vi "Symphony Init.vi"(7 "error In":errorcluster, 9 "Unique id:":string="CCD100", 10 "JYCCDLib.IJYCCDReqd":refnum<k7>) -> (0 "error out":errorcluster, 1 "activeYPixels":i32=256, 2 "activeXPixels":i32=1024, 3 "JYCCDLib.IJYCCDReqd":refnum<k7>, 4 "Name":string="ccd de test", 6 "FirmwareVersion":string="V1.89  CCD_3000")   [LabVIEW 2019]
panel:
  in  "Skip Init":bool
  out "SupportFilesPath":string
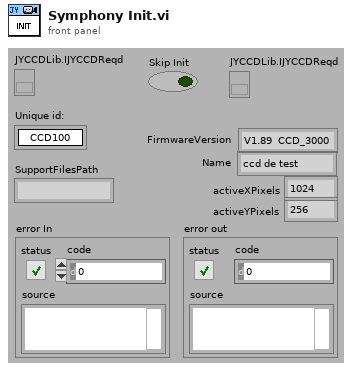
[diagram p1: front panel]
types:
  T1 = enum16{"Open", "Init", "ReadPar", "InitDone", "Error"}
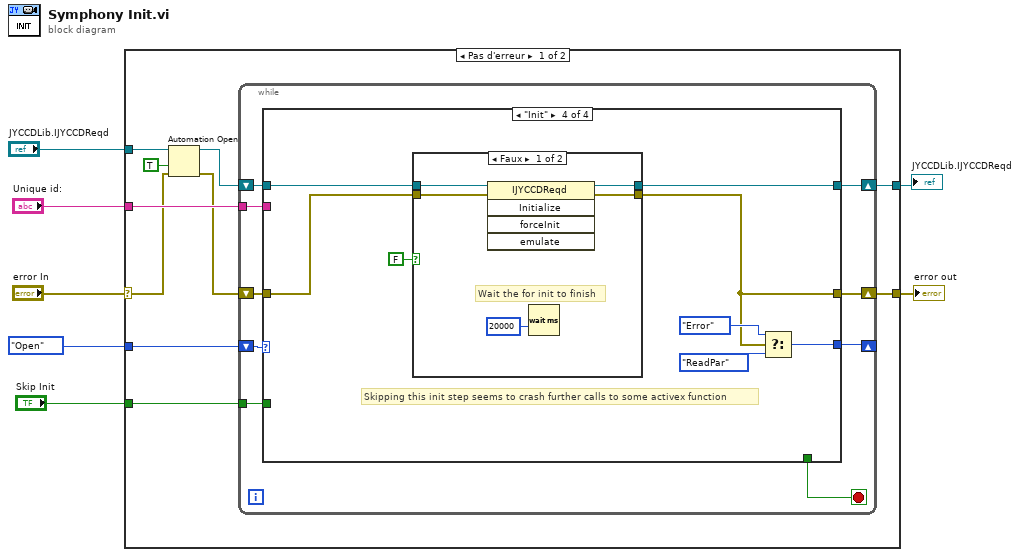
[diagram p0: block diagram]
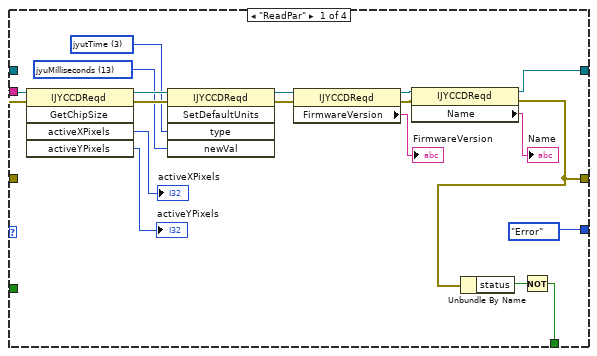
[diagram p2: hidden frame]
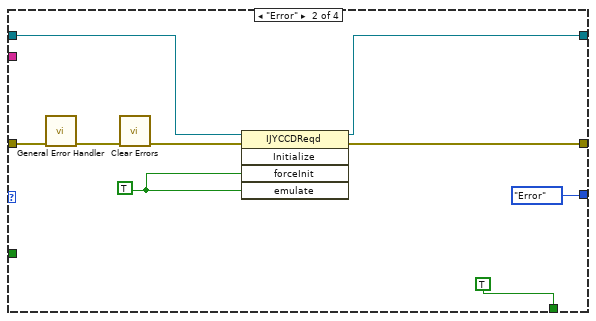
[diagram p3: hidden frame]
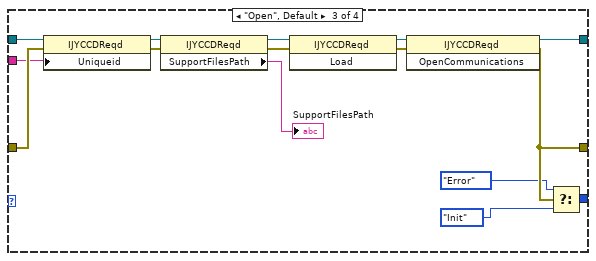
[diagram p4: hidden frame]
diagram:
  n1 = case shown="Pas d'erreur" "error In" {
    selector: "error In" -> [w11 w86]
    tunnel: "Unique id:" -> [w16 _]
    tunnel: "JYCCDLib.IJYCCDReqd" -> [w12 w85]
    tunnel: [w14 w85] -> w5
    tunnel: [w15 w86] -> w4
    tunnel: T1."Open" -> [w17 _]
    tunnel: "Skip Init" -> [w8 _]
    frame No Error {
      n2 = Automation Open(error in (no error)=w11, Automation Refnum=w12, 9:TRUE ("ouvrir une nouvelle instance")) -> (Automation Refnum=w9:refnum<k7>, error out=w10:errorcluster)  [unwired: 1 in]
      n3 = while {
        shift-right: [w22] -> _
        shift-left: w17 -> [w26]
        tunnel: w16 -> [w24]
        shift-right: [w23] -> w15
        shift-left: w10 -> [w25]
        shift-right: [w20] -> w14
        shift-left: w9 -> [w19]
        tunnel: w8 -> [w18]
        stop <- w21 stop-if-true
        n4 = case shown="\"Init\"" w26 {
          tunnel: w19 -> [w33 w48 w55 w76]
          tunnel: w25 -> [w32 w52 w57 w77]
          tunnel: w24 -> [_ _ w56 _]
          tunnel: [w30 w47 w67 w72] -> w23
          tunnel: [T1."Error" T1."Error" w64 w73] -> w22
          tunnel: [w28 TRUE _ _] -> w21
          tunnel: [w27 w46 w58 w71] -> w20
          tunnel: w18 -> [_ _ _ _]
          frame "ReadPar" {
            w41 = 13 items=["jyuUndefined", "jyuMillimeters", "jyuMicrons", "jyuNanometers", "jyuAngstroms", "jyuPicometers", "jyuBandpass", "jyuSteps", "jyuWavenumbers", "jyuDeltaWavenumbers", "jyuElectronVolts", "jyuNanoseconds", "jyuMicroseconds", "jyuMilliseconds", "jyuSeconds", "jyuMinutes", "jyuHours", "jyuVolts", "jyuMillivolts", "jyuMicrovolts", "jyuAmperes", "jyuMilliAmps", "jyuMicroAmps", "jyuCounts", "jyuCountsPerSecond", "jyuDegreesCelcius", "jyuDegreesFahrenheit", "jyuDegreesKelvin", "jyuPixels", "jyuTotalUnitsPlusOne"] ("newVal")
            w40 = 3 items=["jyutUndefined", "jyutWavelength", "jyutSlitWidth", "jyutTime", "jyutTemperature", "jyutDataUnits", "jyutSpatial", "jyutTotalTypesPlusOne"] ("type")
            n5 = invoke class="IJYCCDReqd" method="GetChipSize"(reference=w33, error in=w32) -> (reference out=w42:refnum<k7>, error out=w43:errorcluster, "activeXPixels"=→"activeXPixels":i32, "activeYPixels"=→"activeYPixels":i32)  [unwired: 3 in, 1 out]
            n6 = invoke class="IJYCCDReqd" method="SetDefaultUnits"(reference=w42, error in=w43, "type"=w40, "newVal"=w41) -> (reference out=w44:refnum<k7>, error out=w45:errorcluster)  [unwired: 1 in, 3 out]
            n7 = property class="IJYCCDReqd"(reference=w44, error in=w45) -> (reference out=w37:refnum<k7>, error out=w38:errorcluster, "FirmwareVersion"=→"FirmwareVersion":string)
            n8 = property class="IJYCCDReqd"(reference=w37, error in=w38) -> (reference out=w27:refnum<k7>, error out=w30:errorcluster, "Name"=→"Name":string)
            n9 = Unbundle By Name(w30) -> ("status"=w29:bool)
            n10 = Not(x=w29) -> (.not. x?=w28:bool)
          }
          frame "Error" {
            w50 = TRUE
            n11 = call <vilib>:"General Error Handler.vi"("error in (no error)"=w52) -> ("error out"=w51:errorcluster)  [unwired: 10 in, 4 out]
            n12 = call <vilib>:"Clear Errors.vi"("error in (no error)"=w51) -> ("error out"=w49:errorcluster)  [unwired: 5 in, 1 out]
            n13 = invoke class="IJYCCDReqd" method="Initialize"(reference=w48, error in=w49, "forceInit"=w50, "emulate"=w50) -> (reference out=w46:refnum<k7>, error out=w47:errorcluster)  [unwired: 1 in, 3 out]
          }
          frame "Open", Default {
            n14 = property class="IJYCCDReqd"(reference=w55, error in=w57, "Uniqueid"=w56) -> (reference out=w62:refnum<k7>, error out=w61:errorcluster)
            n15 = property class="IJYCCDReqd"(reference=w62, error in=w61) -> (reference out=w59:refnum<k7>, error out=w60:errorcluster, "SupportFilesPath"=→"SupportFilesPath":string)
            n16 = invoke class="IJYCCDReqd" method="Load"(reference=w59, error in=w60) -> (reference out=w68:refnum<k7>, error out=w69:errorcluster)  [unwired: 1 in, 1 out]
            n17 = invoke class="IJYCCDReqd" method="OpenCommunications"(reference=w68, error in=w69) -> (reference out=w58:refnum<k7>, error out=w67:errorcluster)  [unwired: 1 in, 1 out]
            n18 = Select(t=T1."Error", s=w67, f=T1."Init") -> (s? t:f=w64:T1)
          }
          frame "Init" {
            # "Skipping this init step seems to crash further calls to some activex function"
            n19 = case shown="Faux" FALSE {
              tunnel: w77 -> [w81 w83]
              tunnel: w76 -> [w80 w84]
              tunnel: [w79 w83] -> w72
              tunnel: [w78 w84] -> w71
              frame False {
                # "Wait the for init to finish"
                n20 = invoke class="IJYCCDReqd" method="Initialize"(reference=w80, error in=w81) -> (reference out=w78:refnum<k7>, error out=w79:errorcluster)  [unwired: 3 in, 3 out]
                n21 = Wait (ms)(milliseconds to wait=u32 20000 ("attente (ms)")) -> ()  [unwired: 1 out]
              }
              frame True {
              }
            }
            n22 = Select(t=T1."Error", s=w72, f=T1."ReadPar") -> (s? t:f=w73:T1)
          }
        }
      }
    }
    frame Error {
    }
  }
  "JYCCDLib.IJYCCDReqd" <- w5
  "error out" <- w4
